vi "Get BLISS_Filter Subfolders.vi"(7 "Folder Criteria\n(comma delimited)":string, 8 "error in":errorcluster, 10 "parent path":path) -> (0 "error out":errorcluster, 2 "Valid Paths":path[](array[path]))   [LabVIEW 2020]
uses:
  <vilib>/regexp/Match Regular Expression.xnode
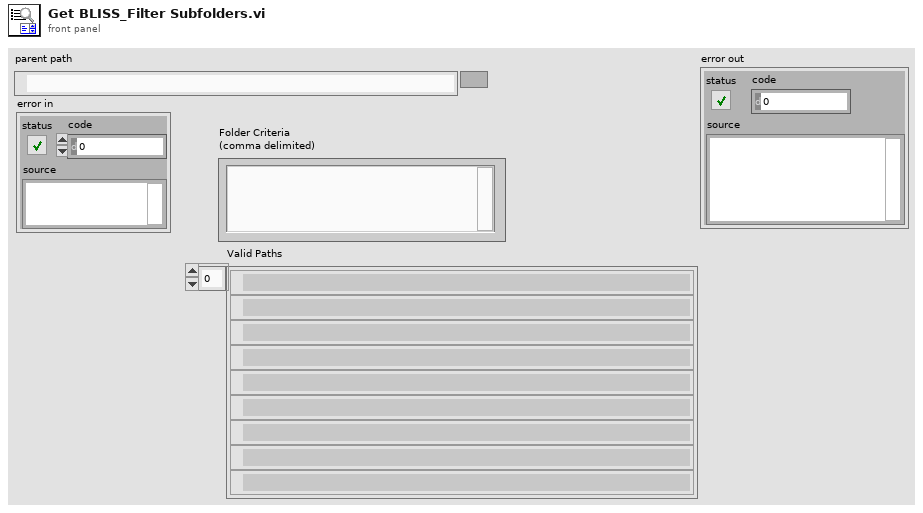
[diagram p1: front panel]
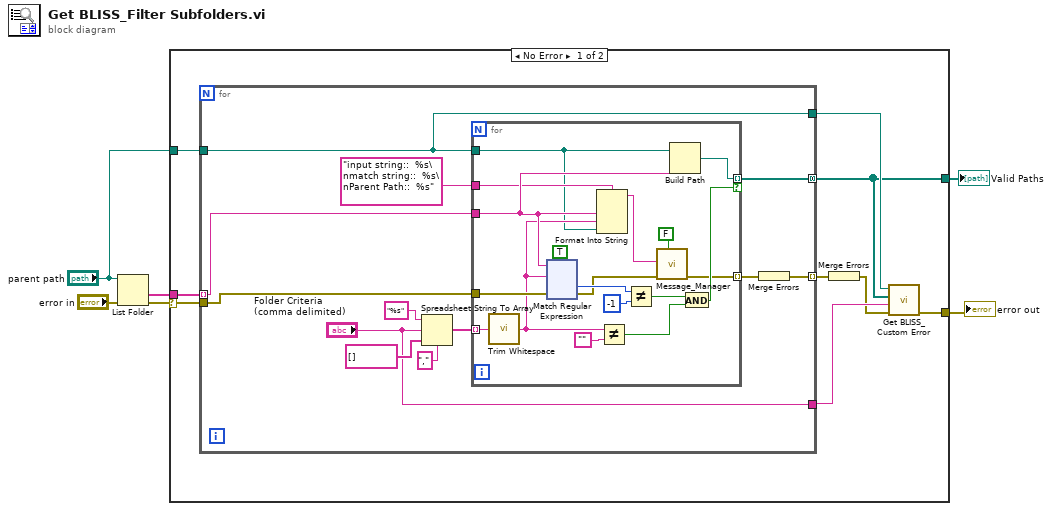
[diagram p0: block diagram]
diagram:
  n1 = List Folder(path="parent path", error in="error in") -> (folder names=w6:string[], error out=w5:errorcluster)  [unwired: 2 in, 2 out]
  n2 = case shown="No Error" w5 {
    selector: w5 -> [w9 w160]
    tunnel: w6 -> [w15 _]
    tunnel: "parent path" -> [w14 _]
    tunnel: [w10 _] -> w2
    tunnel: [w13 w160] -> w1
    frame No Error {
      n3 = for {
        tunnel: w15 -> [w23] mode=indexing
        tunnel: w14 -> [w21]
        tunnel: [w22] -> w10 mode=concatenating
        tunnel: [w21] -> w12
        tunnel: ["Folder Criteria\n(comma delimited)"] -> w11
        tunnel: w9 -> [w20]
        tunnel: [w18] -> w8 mode=indexing
        n4 = Spreadsheet String To Array(delimiter (Tab)=",", format string="%s", spreadsheet string="Folder Criteria\n(comma delimited)", array type (2D Dbl)=string[] []) -> (array=w24:string[])
        n5 = for {
          tunnel: w24 -> [w44] mode=indexing
          tunnel: [w39] -> w22 mode=indexing if=w40
          tunnel: w23 -> [w32]
          tunnel: w21 -> [w28]
          tunnel: w20 -> [w36]
          tunnel: [w34] -> w19 mode=indexing
          tunnel: "input string::  %s\nmatch string::  %s\nParent Path::  %s" ("format string") -> [w29]
          n6 = call <vilib>:"Trim Whitespace.vi"("string"=w44) -> ("trimmed string"=w31:string)  [unwired: 1 in]
          n7 = xnode "Match Regular Expression"("input string"=w32, "regular expression"=w31, "error in"=w36, "ignore case? (F)"=TRUE) -> ("offset past match"=w37:i32, "error out"=w35:errorcluster)  [unwired: 2 in, 3 out]
          n8 = Format Into String(format string=w29, w32, w31, w28) -> (resulting string=w30:string)  [unwired: 2 in, 1 out]
          n9 = Not Equal?(x=w31, y="") -> (x != y?=w41:bool)
          n10 = Not Equal?(x=w37, y=-1) -> (x != y?=w42:bool)
          n11 = call "Message_Manager.vi"("Log only on Err"=FALSE ("Force Log Entry (T)"), "error in"=w35, "New Entry"=w30) -> ("error out"=w34:errorcluster)  [unwired: 3 in, 5 out]
          n12 = Build Path(base path=w28, name or relative path=w32) -> (appended path=w39:path)
          n13 = And(x=w42, y=w41) -> (x .and. y?=w40:bool)
        }
        n14 = Merge Errors(w19) -> (w18:errorcluster)
      }
      n15 = Merge Errors(w8) -> (w7:errorcluster)
      n16 = call "Get BLISS_Custom Error.vi"("error in (no error)"=w7, "search criteria"=w11, "Array"=w10, "Parent path"=w12) -> ("error out"=w13:errorcluster)  [unwired: 7 in]
    }
    frame Error {
    }
  }
  "error out" <- w1
  "Valid Paths" <- w2
